vi "DAQmx quick buffer update.vi"() -> ()   [LabVIEW 2012]
uses:
  <vilib>/Utility/error.llb/DialogType.ctl
  <vilib>/DAQmx/write.llb/DAQmx Write (Analog Wfm 1Chan NSamp).vi
  <vilib>/DAQmx/create/channels.llb/DAQmx Create Channel (AO-Voltage-Basic).vi
  <vilib>/DAQmx/configure/timing.llb/DAQmx Timing (Sample Clock).vi
  <vilib>/DAQmx/miscellaneous.llb/DAQmx Fill In Error Info.vi
  <vilib>/measure/NI_MABase.lvlib
  <resource>/objmgr/daqmx.rc
panel:
  in  "Blocks":i32=2
  out "Output.OnbrdBufSize":u32
  out "Output.BufSize":u32
  out "Offset":i32
  out "RelativeTo":i32(ring)=10424 items=["First Sample"=10424, "Current Write Position"=10430]
  out "TotalSampPerChanGenerated":dbl
  out "CurrWritePos":dbl
  out "SpaceAvail":u32
  out "Waveform Graph":waveform(dbl)(graph)
  in  "stop":bool
  in  "Samples in buffer":dbl=1000.0
  in  "rate":dbl=1000.0
  in  "amplitude":dbl=1.0 format="%0.2p"
  in  "frequency":dbl=10.0 format="%0.2p"
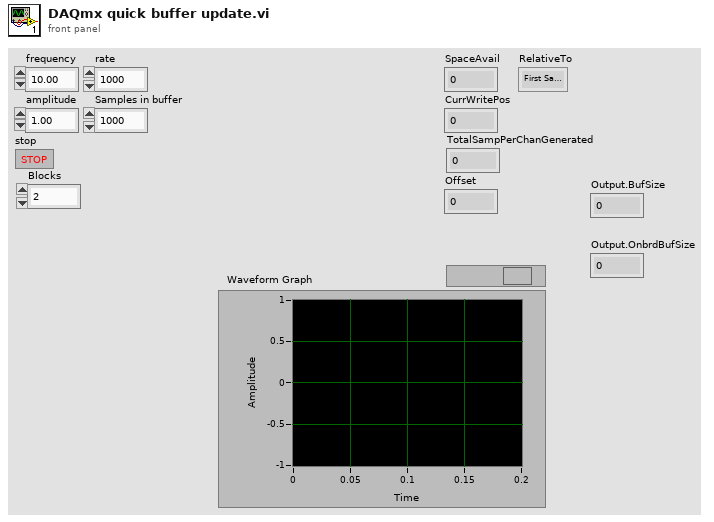
[diagram p1: front panel]
types:
  T1 = typedef "DialogType.ctl" = u16
  T2 = enum16{"Sine Wave", "Triangle Wave", "Square Wave", "Sawtooth Wave"}
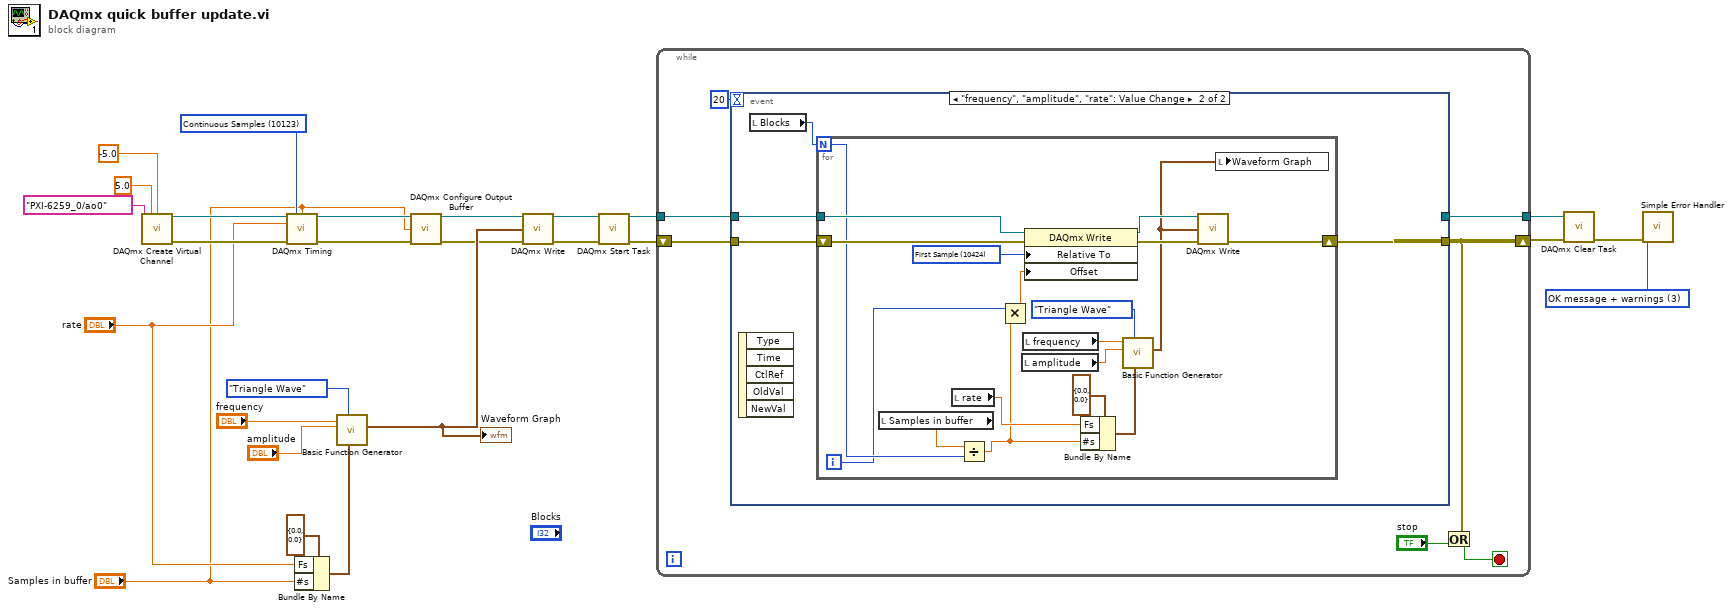
[diagram p0: block diagram]
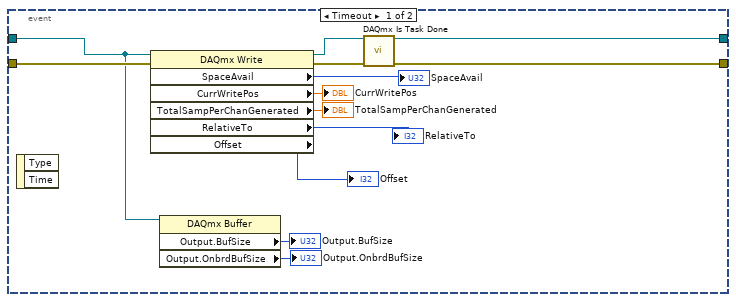
[diagram p2: hidden frame]
diagram:
  w8 = T1 3 items=["no dialog", "OK message", "continue or stop message", "OK message + warnings", "continue/stop + warnings"] ("type of dialog (OK msg:1)")
  w21 = 10123 items=["Finite Samples"=10178, "Continuous Samples"=10123, "Hardware Timed Single Point"=12522] ("sample mode")
  n1 = call-poly <vilib>:"DAQmx Create Virtual Channel.vi"("maximum value"=5.0, "minimum value"=-5.0, "physical channels"=tag "PXI-6259_0/ao0") -> ("task out"=w22:refnum<k21>, "error out"=w23:errorcluster)  [unwired: 11 in]
  n2 = call-poly <vilib>:"DAQmx Timing.vi"("task/channels in"=w22, "sample mode"=w21, "samples per channel"="Samples in buffer", "rate"="rate", "error in"=w23) -> ("task out"=w5:refnum<k21>, "error out"=w4:errorcluster)  [unwired: 9 in]
  n3 = Bundle By Name(cluster=cluster{"Fs":dbl, "#s":dbl} {"Fs"=0.0, "#s"=0.0} ("sampling info"), "Fs"="rate", "#s"="Samples in buffer") -> (w16:cluster{"Fs":dbl, "#s":dbl})
  n4 = call <vilib>:"Basic Function Generator.vi"("sampling info"=w16, "signal type"=T2."Triangle Wave", "amplitude"="amplitude", "frequency"="frequency") -> ("signal out"=w7:waveform(dbl))  [unwired: 5 in, 2 out]
  "Waveform Graph" <- w7
  n5 = call <vilib>:"DAQmx Configure Output Buffer.vi"("task/channels in"=w5, "buffer size (in samples per channel)"="Samples in buffer", "error in"=w4) -> ("task out"=w1:refnum<k21>, "error out"=w3:errorcluster)  [unwired: 11 in]
  n6 = call-poly <vilib>:"DAQmx Write.vi"("task/channels in"=w1, "data"=w7, "error in"=w3) -> ("task out"=w6:refnum<k21>, "error out"=w14:errorcluster)  [unwired: 10 in, 1 out]
  n7 = call <vilib>:"DAQmx Start Task.vi"("task/channels in"=w6, "error in"=w14) -> ("task out"=w13:refnum<k21>, "error out"=w12:errorcluster)  [unwired: 12 in]
  n8 = while {
    tunnel: w13 -> [w30]
    shift-right: [w28] -> w11
    shift-left: w12 -> [w31]
    tunnel: [w29] -> w10
    stop <- w32 stop-if-true
    n9 = event shown="[1] \"frequency\", \"amplitude\", \"rate\": Value Change" {
      selector: _ -> [_ _]
      dyn-events: _ -> [_ _]
      timeout: 20 -> [_ _]
      tunnel: w31 -> [w44 w50]
      tunnel: w30 -> [w36 w49]
      tunnel: [w46 w48] -> w28
      tunnel: [w45 _] -> w29
      event Timeout {
        n10 = event-data() -> ()  [unwired: 1 in, 2 out]
        n11 = property class="DAQmx Write"(reference=w36, error in=w44) -> (reference out=w43:refnum<k21>, error out=w42:errorcluster, "SpaceAvail"=→"SpaceAvail":u32, "CurrWritePos"=→"CurrWritePos":dbl, "TotalSampPerChanGenerated"=→"TotalSampPerChanGenerated":dbl, "RelativeTo"=→"RelativeTo":i32, "Offset"=→"Offset":i32)
        n12 = property class="DAQmx Buffer"(reference=w36) -> ("Output.BufSize"=→"Output.BufSize":u32, "Output.OnbrdBufSize"=→"Output.OnbrdBufSize":u32)  [unwired: 1 in, 2 out]
        n13 = call <vilib>:"DAQmx Is Task Done.vi"("task/channels in"=w43, "error in"=w42) -> ("task out"=w45:refnum<k21>, "error out"=w46:errorcluster)  [unwired: 11 in, 1 out]
      }
      event "frequency", "amplitude", "rate": Value Change {
        n14 = event-data() -> ()  [unwired: 1 in, 5 out]
        n15 = local read "Blocks"() -> (w47:i32)
        n16 = for {
          N: w47 -> [w54]
          tunnel: w49 -> [w64]
          shift-right: [w55] -> w48
          shift-left: w50 -> [w65]
          i -> [w52]
          w61 = 10424 items=["First Sample"=10424, "Current Write Position"=10430] ("RelativeTo")
          n17 = local read "Samples in buffer"() -> (w57:dbl)
          n18 = local read "rate"() -> (w58:dbl)
          n19 = Divide(x=w57, y=w54) -> (x/y=w51:dbl)
          n20 = Multiply(x=w52, y=w51) -> (x*y=w53:dbl)
          n21 = local read "amplitude"() -> (w66:dbl)
          n22 = local read "frequency"() -> (w67:dbl)
          n23 = property class="DAQmx Write"(reference=w64, error in=w65, "Relative To"=w61, "Offset"=w53) -> (reference out=w63:refnum<k21>, error out=w62:errorcluster)
          n24 = Bundle By Name(cluster=cluster{"Fs":dbl, "#s":dbl} {"Fs"=0.0, "#s"=0.0} ("sampling info"), "Fs"=w58, "#s"=w51) -> (w59:cluster{"Fs":dbl, "#s":dbl})
          n25 = call <vilib>:"Basic Function Generator.vi"("sampling info"=w59, "signal type"=T2."Triangle Wave", "amplitude"=w66, "frequency"=w67) -> ("signal out"=w56:waveform(dbl))  [unwired: 5 in, 2 out]
          n26 = call-poly <vilib>:"DAQmx Write.vi"("task/channels in"=w63, "data"=w56, "error in"=w62) -> ("error out"=w55:errorcluster)  [unwired: 10 in, 2 out]
          n27 = local write "Waveform Graph"(w56) -> ()
        }
      }
    }
    n28 = Or(x=w28, y="stop") -> (x .or. y?=w32:bool)
  }
  n29 = call <vilib>:"DAQmx Clear Task.vi"("task in"=w10, "error in"=w11) -> ("error out"=w9:errorcluster)  [unwired: 13 in]
  n30 = call <vilib>:"Simple Error Handler.vi"("type of dialog (OK msg:1)"=w8, "error in (no error)"=w9) -> ()  [unwired: 3 in, 5 out]
